vi "EncodeUnsignedHundredths.vi"(1 "Data In":dbl[](array[numeric])) -> (0 "Data Out":u8[](array[numeric]))   [LabVIEW 2014, in "navX-MXP IMU.lvlib"]
uses:
  navX-MXP IMU.lvlib
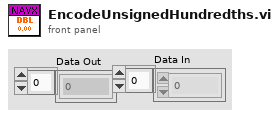
[diagram p1: front panel]
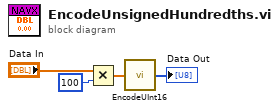
[diagram p0: block diagram]
diagram:
  n1 = Multiply(x="Data In", y=100) -> (x*y=w2:dbl[])
  n2 = call "EncodeUInt16.vi"("Data In"=w2) -> ("Data Out"=→"Data Out":u8[])
